vi "LSMcontroller_v62_updatedpointscan.vi"() -> ()   [LabVIEW 2015] (continued)
                            n96 = call "createdatafolder.vi"("timestamp in"=w2092) -> ("current data path"=w2093:path, "timestamp out"=w2091:timestamp)
                            n97 = local write "data dir"(w2093) -> ()
                          }
                        }
                        n98 = stacked-sequence {
                          tunnel: w2088 -> [_ w2100 _ _ _ _ _ _ _ _]
                          tunnel: [_ _ _ _ _ w2243 _ _ _ _] -> w2086
                          tunnel: [_ _ _ _ _ w2242 _ _ _ _] -> w2085
                          tunnel: [_ _ _ _ _ w2241 _ _ _ _] -> w2084
                          tunnel: [_ _ _ _ _ w2240 _ _ _ _] -> w2083
                          tunnel: [_ _ _ _ _ w2239 _ _ _ _] -> w2082
                          tunnel: [_ _ _ _ _ w2238 _ _ _ _] -> w2081
                          tunnel: [_ _ _ _ _ w2237 _ _ _ _] -> w2080
                          tunnel: [_ _ _ _ _ w2236 _ _ _ _] -> w2079
                          tunnel: [_ _ _ _ _ w2235 _ _ _ _] -> w2078
                          tunnel: [_ _ _ _ _ w2234 _ _ _ _] -> w2077
                          tunnel: [_ _ _ _ _ w2233 _ _ _ _] -> w2076
                          tunnel: [_ _ _ _ _ w2232 _ _ _ _] -> w2075
                          tunnel: [_ _ _ _ _ w2231 _ _ _ _] -> w2074
                          tunnel: [_ _ _ _ _ w2230 _ _ _ _] -> w2073
                          frame #0 {
                            n99 = local read "AI channels"() -> (w2099:i32[])
                            n100 = local read "CI channels"() -> (w2098:i32[])
                            n101 = call "2pparameters.vi"("command"="get") -> ("params out"=w2096:T10)  [unwired: 1 in]
                            n102 = Bundle By Name(cluster=w2096, "aAI"=w2099, "aCI"=w2098) -> (w2097:T10)
                            n103 = call "2pparameters.vi"("Params in"=w2097, "command"="set") -> ()  [unwired: 1 out]
                          }
                          frame #1 {
                            n104 = local read "Vy-min ref"() -> (w2104:dbl)
                            n105 = local read "Vy-max ref"() -> (w2105:dbl)
                            n106 = local read "Angle ref"() -> (w2103:dbl)
                            n107 = local read "Vx-min ref"() -> (w2106:dbl)
                            n108 = local write "counts"(0 ("counts")) -> ()
                            n109 = local write "graphtab"(T5."image" ("graphtab")) -> ()
                            n110 = local read "Vx-max ref"() -> (w2107:dbl)
                            n111 = property on="Stop" class="Bool (strict)"("Visible"=TRUE, "DisabledEnum"=T7."Enabled" ("Disabled")) -> ()  [unwired: 2 in, 2 out]
                            n112 = property on="Start" class="Bool (strict)"("Visible"=FALSE, "DisabledEnum"=T7."Disabled and Grayed Out" ("Disabled")) -> ()  [unwired: 2 in, 2 out]
                            n113 = script code="Xic=(ximax+ximin)./2;\nYic=(yimax+yimin)./2;\nximin=ximin-Xic;\nymin=ymin-Yic;\nxirmin=ximin.*cos(pi/180.*phi)+yimin.*sin(pi./180.*phi)+Xic;\nyirmin=-ximin.*sin(pi./180.*phi)+yimin.*cos(pi./180.*phi)+Yic;"("ximax"=w2107, "ximin"=w2106, "yimax"=w2105, "yimin"=w2104, "phi"=w2103) -> ("xirmin"=w2102:dbl, "yirmin"=w2101:dbl)  [unwired: 1 in, 1 out]
                            n114 = stacked-sequence {
                              tunnel: w2100 -> [_ w2132 _]
                              frame #0 {
                                n115 = local read "Measurement"() -> (w2114:T4)
                                n116 = case shown="\"X-Y-Z stack\"" w2114 {
                                frame "X-Y-t movie", Default {
                                n117 = call "2pparameters.vi"("command"="get") -> ("params out"=w2117:T10)  [unwired: 1 in]
                                n118 = Bundle By Name(cluster=w2117, "type"="X-Y-t movie") -> (w2115:T10)
                                n119 = call "2pparameters.vi"("Params in"=w2115, "command"="set") -> ()  [unwired: 1 out]
                                }
                                frame "X-Y-Z stack" {
                                n120 = call "2pparameters.vi"("command"="get") -> ("params out"=w2122:T10)  [unwired: 1 in]
                                n121 = Bundle By Name(cluster=w2122, "type"="X-Y-Z stack") -> (w2120:T10)
                                n122 = call "2pparameters.vi"("Params in"=w2120, "command"="set") -> ()  [unwired: 1 out]
                                }
                                frame "Lifetime (scan)" {
                                n123 = call "2pparameters.vi"("command"="get") -> ("params out"=w2127:T10)  [unwired: 1 in]
                                n124 = Bundle By Name(cluster=w2127, "type"="Lifetime (scan)") -> (w2125:T10)
                                n125 = call "2pparameters.vi"("Params in"=w2125, "command"="set") -> ()  [unwired: 1 out]
                                }
                                }
                              }
                              frame #1 {
                                n126 = Format Date/Time String(time format string (%c)="%Y%m%d", seconds (now)=w2132) -> (date/time string=w2131:string)  [unwired: 1 in]
                                n127 = Format Date/Time String(time format string (%c)="%H%M%S", seconds (now)=w2132) -> (date/time string=w2130:string)  [unwired: 1 in]
                                n128 = call "2pparameters.vi"("command"="get") -> ("params out"=w2136:T10)  [unwired: 1 in]
                                n129 = Bundle By Name(cluster=w2136, "date"=w2131, "time"=w2130) -> (w2135:T10)
                                n130 = call "2pparameters.vi"("Params in"=w2135, "command"="set") -> ()  [unwired: 1 out]
                              }
                              frame #2 {
                                n131 = call "configuration.vi"("command"="get") -> ("config out"=w2146:T11)  [unwired: 2 in, 1 out]
                                n132 = Unbundle By Name(w2146) -> ("CI names"=w2147:string[], "AI names"=w2148:string[])
                                n133 = call "2pparameters.vi"("command"="get") -> ("params out"=w2142:T10)  [unwired: 1 in]
                                n134 = Unbundle By Name(w2142) -> ("aCI"=w2143:i32[], "aAI"=w2144:i32[])
                                n135 = for {
                                tunnel: w2143 -> [w2158] mode=indexing
                                tunnel: w2147 -> [w2159]
                                tunnel: [w2157] -> w2149 mode=indexing
                                n136 = Index Array(array=w2159, index=w2158) -> (element=w2157:string)
                                }
                                n137 = for {
                                tunnel: w2144 -> [w2155] mode=indexing
                                tunnel: w2148 -> [w2156]
                                tunnel: [w2154] -> w2150 mode=indexing
                                n138 = Index Array(array=w2156, index=w2155) -> (element=w2154:string)
                                }
                                n139 = Build Array (concatenate)(w2149, w2150) -> (w2140:string[])
                                n140 = for {
                                tunnel: w2140 -> [w2152] mode=indexing
                                tunnel: [w2151] -> w2139 mode=indexing
                                i -> [w2153]
                                n141 = Bundle("String"=w2152, w2153) -> (w2151:cluster{"String":string, i32})  [unwired: 1 in]
                                }
                                n142 = property on="image1list" class="Ring (strict)"("StringsAndValues[]"=w2139) -> ()  [unwired: 2 in, 2 out]
                                n143 = property on="image2list" class="Ring (strict)"("StringsAndValues[]"=w2139) -> ()  [unwired: 2 in, 2 out]
                              }
                            }
                            n144 = call "setposition.vi"("Vy"=w2101, "Vx"=w2102) -> ()  [unwired: 1 in]
                          }
                          frame #2 {
                            n145 = call "X-array-databuffer.vi"("command"=enum16{"get", "set", "clear", "append"}."clear") -> ()  [unwired: 3 in, 2 out]
                            n146 = call "Y-array-databuffer.vi"("command"=enum16{"get", "set", "clear", "append"}."clear") -> ()  [unwired: 3 in, 2 out]
                            n147 = call "2pparameters.vi"("command"="get") -> ("params out"=w2162:T10)  [unwired: 1 in]
                            n148 = Unbundle By Name(w2162) -> ("autoshutter"=w2163:bool, "auto OD"=w2160:bool)
                            n149 = call "allAI-temp_img.vi"("command"=enum16{"get", "set", "clear", "append"}."clear") -> ()  [unwired: 3 in, 2 out]
                            n150 = case shown="True" w2160 {
                              frame False {
                              }
                              frame True {
                                n151 = call "configuration.vi"("command"="get") -> ("config out"=w2171:T11)  [unwired: 2 in, 1 out]
                                n152 = Unbundle By Name(w2171) -> ("image OD"=w2172:u16)
                                n153 = local read "ODfilt"() -> (w2169:u16)
                                n154 = call "filterwheelcontrol_nothorlabslib.vi"("Current OD filt"=w2169, "New ODfilt"=w2172) -> ()  [unwired: 1 in]
                              }
                            }
                            n155 = case shown="True" w2163 {
                              frame False {
                              }
                              frame True {
                                n156 = call "shuttercontrol.vi"("command"="close") -> ()  [unwired: 1 in, 1 out]
                              }
                            }
                            n157 = call "CH1-temp.vi"("command"=enum16{"get", "set", "clear", "add row"}."clear") -> ()  [unwired: 3 in, 2 out]
                            n158 = call "CH2-temp.vi"("command"=enum16{"get", "set", "clear", "add row"}."clear") -> ()  [unwired: 3 in, 2 out]
                          }
                          frame #3 {
                            n159 = local read "avpp"() -> (w2206:i32)
                            n160 = local read "Angle ref"() -> (w2205:dbl)
                            n161 = local read "ROI Type"() -> (w2204:u16)
                            n162 = local read "xpixels ref"() -> (w2201:i32)
                            n163 = local read "Vx-min ref"() -> (w2200:dbl)
                            n164 = local read "Vx-max ref"() -> (w2199:dbl)
                            n165 = local read "ypixels ref"() -> (w2197:i32)
                            n166 = local read "Vy-min ref"() -> (w2198:dbl)
                            n167 = local read "Vy-max ref"() -> (w2194:dbl)
                            n168 = local read "Sampling rate"() -> (w2188:dbl)
                            n169 = local read "finite samples"() -> (w2189:bool)
                            n170 = local read "continuous"() -> (w2192:bool)
                            n171 = local read "wavdet"() -> (w2193:bool)
                            n172 = local read "# of frames"() -> (w2191:i32)
                            n173 = local read "maxbufferAI"() -> (w2190:i32)
                            n174 = local read "Override AI buffer"() -> (w2174:bool)
                            n175 = call "2pparameters.vi"("command"="get") -> ("params out"=w2203:T10)  [unwired: 1 in]
                            n176 = Bundle By Name(cluster=w2203, "avpp"=w2206, "Angle Img"=w2205, "Xpixels Img"=w2201, "Vx-min Img"=w2200, "VX-max Img"=w2199, "Ypixels Img"=w2197, "Vy-min Img"=w2198, "Vy-max Img"=w2194, "srate"=w2188, "srate Img"=w2188, "finite"=w2189, "cont"=w2192, "wavdet"=w2193, "measpoints"=w2191, "maxbufferAI"=w2190, "Drawing Mode"=w2204, "Vz-reset"=0.0, "AIoverride"=w2174) -> (w2195:T10)
                            n177 = call "2pparameters.vi"("Params in"=w2195, "command"="set") -> ()  [unwired: 1 out]
                            n178 = local read "Vholding (mV)"() -> (w2177:sgl)
                            n179 = local read "Current Clamp"() -> (w2183:bool)
                            n180 = local read "Voltage Clamp"() -> (w2182:bool)
                            n181 = local read "OCgain"() -> (w2178:sgl)
                            n182 = local read "CC_ICgain"() -> (w2181:dbl)
                            n183 = local read "holdon"() -> (w2176:bool)
                            n184 = call "patchparameters.vi"("command"="get") -> ("Params out"=w2185:T13)  [unwired: 1 in]
                            n185 = Bundle By Name(cluster=w2185, "VC"=w2182, "CC"=w2183, "CC_icg (pA/mv)"=w2181, "VC_icg (mV/mV)"=sgl 10.0, "OCG (mV/pA)"=w2178, "OVG (mV/mV)"=0.1, "Vhold (mV)"=w2177, "holdon"=w2176) -> (w2184:T13)
                            n186 = call "patchparameters.vi"("Params in"=w2184, "command"="set") -> ()  [unwired: 1 out]
                          }
                          frame #4 {
                            # "Generate Waveforms for Scanning Mirrors"
                            n187 = call "2pparameters.vi"("command"="get") -> ("params out"=w2221:T10)  [unwired: 1 in]
                            n188 = Unbundle By Name(w2221) -> ("srate Img"=w2220:sgl, "Angle Img"=w2219:dbl, "VX-max Img"=w2218:dbl, "Vx-min Img"=w2217:dbl, "Xpixels Img"=w2216:i32, "Ypixels Img"=w2215:i32, "Vy-max Img"=w2214:dbl, "Vy-min Img"=w2213:dbl, "Drawing Mode"=w2212:u16)
                            n189 = call "ROI-databuffer.vi"("command"=enum16{"get", "set", "clear", "append"}."get") -> ("array out"=w2211:cluster{"x":sgl, "y":sgl}[])  [unwired: 4 in]
                            n190 = call "ScanningWaveform_v4.vi"("Vy-min"=w2213, "Vy-max"=w2214, "yPixels/tPixels"=w2215, "xPixels/rPixels"=w2216, "Vx-min"=w2217, "Vx-max"=w2218, "Drawing Mode"=w2212, "Angle"=w2219, "AOrate"=w2220, "Points"=w2211) -> ("numPixels"=w2207:dbl, "Y-WaveArray"=w2210:dbl[], "P"=w2208:dbl, "X-WaveArray"=w2209:dbl[])  [unwired: 6 in]
                            n191 = call "2pparameters.vi"("command"="get") -> ("params out"=w2229:T10)  [unwired: 1 in]
                            n192 = call "Y-array-databuffer.vi"("array in"=w2210, "command"=enum16{"get", "set", "clear", "append"}."set") -> ()  [unwired: 2 in, 2 out]
                            n193 = call "X-array-databuffer.vi"("array in"=w2209, "command"=enum16{"get", "set", "clear", "append"}."set") -> ()  [unwired: 2 in, 2 out]
                            n194 = Bundle By Name(cluster=w2229, "P"=w2208, "sAOxy"=w2207) -> (w2226:T10)
                            n195 = call "2pparameters.vi"("Params in"=w2226, "command"="set") -> ()  [unwired: 1 out]
                          }
                          frame #5 {
                            # "rem2Ps"
                            # "A2Ps"
                            # "Al"
                            # "Rl"
                            n196 = stacked-sequence {
                              seq-local: [w2248 _ _ _ _ _ _ _ _ _ _] -> [_ w2360 _ w2415 _ w2495 _ _ _ _ _]
                              seq-local: [w2249 _ _ _ _ _ _ _ _ _ _] -> [_ w2361 w2371 _ w2464 _ _ _ _ _ _]
                              seq-local: [_ _ w2370 _ _ _ _ _ _ _ _] -> [_ _ _ _ w2458 _ _ _ _ _ _]
                              seq-local: [_ _ _ w2414 _ _ _ _ _ _ _] -> [_ _ _ _ _ w2494 _ _ _ _ _]
                              seq-local: [w2245 _ _ _ _ _ _ _ _ _ _] -> [_ w2357 _ _ _ _ _ _ w2680 w2748 _]
                              seq-local: [w2244 _ _ _ _ _ _ _ _ _ _] -> [_ w2356 _ _ _ _ _ _ w2681 w2749 _]
                              seq-local: [w2251 _ _ _ _ _ _ _ _ _ _] -> [_ _ _ _ _ _ w2533 _ w2679 w2747 _]
                              seq-local: [w2247 _ _ _ _ _ _ _ _ _ _] -> [_ w2355 _ _ _ _ w2532 w2600 _ _ _]
                              seq-local: [w2246 _ _ _ _ _ _ _ _ _ _] -> [_ w2354 _ _ _ _ w2531 w2599 _ _ _]
                              seq-local: [w2250 _ _ _ _ _ _ _ _ _ _] -> [_ _ _ _ _ _ w2530 w2598 _ _ _]
                              tunnel: [_ _ w2369 _ _ _ _ _ _ _ _] -> w2242
                              tunnel: [_ _ w2368 _ _ _ _ _ _ _ _] -> w2241
                              tunnel: [w2249 _ _ _ _ _ _ _ _ _ _] -> w2243
                              tunnel: [w2248 _ _ _ _ _ _ _ _ _ _] -> w2240
                              tunnel: [_ _ _ w2413 _ _ _ _ _ _ _] -> w2239
                              tunnel: [_ _ _ w2412 _ _ _ _ _ _ _] -> w2238
                              tunnel: [w2247 _ _ _ _ _ _ _ _ _ _] -> w2237
                              tunnel: [w2246 _ _ _ _ _ _ _ _ _ _] -> w2236
                              tunnel: [_ _ _ _ _ _ w2529 _ _ _ _] -> w2235
                              tunnel: [_ _ _ _ _ _ _ w2597 _ _ _] -> w2234
                              tunnel: [w2245 _ _ _ _ _ _ _ _ _ _] -> w2233
                              tunnel: [w2244 _ _ _ _ _ _ _ _ _ _] -> w2232
                              tunnel: [_ _ _ _ _ _ _ _ w2678 _ _] -> w2231
                              tunnel: [_ _ _ _ _ _ _ _ _ w2746 _] -> w2230
                              frame #0 {
                                # "for a next version, give ome thought to\nthe possibilit of intermittently updating the\nwaveforms. it will have to be a calculation\nbased on speed of CPU and program on the one hand\nand length of measurement on the other. but then it should be possible, in principle, to \nupdate the waveform on the fly and that way cut up a longer measurement in smaller parts."
                                # "Y"
                                # "X"
                                n197 = stacked-sequence {
                                tunnel: [w2252 _ _ _] -> w2249
                                tunnel: [_ w2264 _ _] -> w2248
                                tunnel: [_ _ _ w2321] -> w2244
                                tunnel: [_ _ _ w2320] -> w2245
                                tunnel: [_ _ _ w2319] -> w2251
                                tunnel: [_ _ w2279 _] -> w2247
                                tunnel: [_ _ w2278 _] -> w2246
                                tunnel: [_ _ w2277 _] -> w2250
                                frame #0 {
                                n198 = call "configuration.vi"("command"="get") -> ("config out"=w2254:T11)  [unwired: 2 in, 1 out]
                                n199 = Unbundle By Name(w2254) -> ("Voltage to Xgalvo"=w2253:i32)
                                n200 = call "2pparameters.vi"("command"="get") -> ("params out"=w2258:T10)  [unwired: 1 in]
                                n201 = in-place {
                                in-place-border: w2253 -> [w2263]
                                in-place-border: [w2260] -> w2252
                                n202 = in-place-cluster #1(w2258) -> ("aAO"=w2262:u32[])
                                n203 = call "add channel to active arrayv2.vi"("line array in"=w2262, "line to add"=w2263) -> ("line array out"=w2261:u32[], "addition"=w2260:bool)  [unwired: 1 out]
                                n204 = in-place-cluster #1("aAO"=w2261) -> (w2256:T10)
                                }
                                n205 = call "2pparameters.vi"("Params in"=w2256, "command"="set") -> ()  [unwired: 1 out]
                                }
                                frame #1 {
                                n206 = call "configuration.vi"("command"="get") -> ("config out"=w2266:T11)  [unwired: 2 in, 1 out]
                                n207 = Unbundle By Name(w2266) -> ("Voltage to Ygalvo"=w2265:i32)
                                n208 = call "2pparameters.vi"("command"="get") -> ("params out"=w2270:T10)  [unwired: 1 in]
                                n209 = in-place {
                                in-place-border: w2265 -> [w2275]
                                in-place-border: [w2272] -> w2264
                                n210 = in-place-cluster #2(w2270) -> ("aAO"=w2274:u32[])
                                n211 = call "add channel to active arrayv2.vi"("line array in"=w2274, "line to add"=w2275) -> ("line array out"=w2273:u32[], "addition"=w2272:bool)  [unwired: 1 out]
                                n212 = in-place-cluster #2("aAO"=w2273) -> (w2268:T10)
                                }
                                n213 = call "2pparameters.vi"("Params in"=w2268, "command"="set") -> ()  [unwired: 1 out]
                                }
                                frame #2 {
                                n214 = call "2pparameters.vi"("command"="get") -> ("params out"=w2281:T10)  [unwired: 1 in]
                                n215 = Unbundle By Name(w2281) -> ("autoshutter"=w2280:bool, "wavdet"=w2276:bool)
                                n216 = case shown="True" w2280 {
                                tunnel: [w2286 w2306] -> w2279
                                tunnel: [w2285 FALSE ("removal")] -> w2278
                                tunnel: [w2284 w2304] -> w2277
                                tunnel: w2276 -> [w2283 _]
                                frame False {
                                n217 = case shown="False" w2283 {
                                tunnel: [FALSE ("addition") FALSE ("addition")] -> w2286
                                tunnel: [w2288 FALSE ("removal")] -> w2285
                                tunnel: [w2287 _] -> w2284
                                frame False {
                                n218 = call "configuration.vi"("command"="get") -> ("config out"=w2294:T11)  [unwired: 2 in, 1 out]
                                n219 = Unbundle By Name(w2294) -> ("2P shutter"=w2291:i32)
                                n220 = call "2pparameters.vi"("command"="get") -> ("params out"=w2292:T10)  [unwired: 1 in]
                                n221 = in-place {
                                in-place-border: w2291 -> [w2301]
                                in-place-border: [w2298] -> w2288
                                in-place-border: [w2297] -> w2287
                                n222 = in-place-cluster #3(w2292) -> ("aDO"=w2300:u32[])
                                n223 = call "remove channel from active arrayv2.vi"("line array in"=w2300, "line to remove"=w2301) -> ("line array out"=w2299:u32[], "removal"=w2298:bool, "index"=w2297:i32)
                                n224 = in-place-cluster #3("aDO"=w2299) -> (w2289:T10)
                                }
                                n225 = call "2pparameters.vi"("Params in"=w2289, "command"="set") -> ()  [unwired: 1 out]
                                }
                                frame True {
                                }
                                }
                                }
                                frame True {
                                n226 = call "configuration.vi"("command"="get") -> ("config out"=w2308:T11)  [unwired: 2 in, 1 out]
                                n227 = call "2pparameters.vi"("command"="get") -> ("params out"=w2312:T10)  [unwired: 1 in]
                                n228 = Unbundle By Name(w2308) -> ("2P shutter"=w2307:i32)
                                n229 = in-place {
                                in-place-border: w2307 -> [w2318]
                                in-place-border: [w2315] -> w2306
                                in-place-border: [w2314] -> w2304
                                n230 = in-place-cluster #4(w2312) -> ("aDO"=w2317:u32[])
                                n231 = call "add channel to active arrayv2.vi"("line array in"=w2317, "line to add"=w2318) -> ("line array out"=w2316:u32[], "addition"=w2315:bool, "index"=w2314:i32)
                                n232 = in-place-cluster #4("aDO"=w2316) -> (w2310:T10)
                                }
                                n233 = call "2pparameters.vi"("Params in"=w2310, "command"="set") -> ()  [unwired: 1 out]
                                }
                                }
                                }
                                frame #3 {
                                n234 = local read "Measurement"() -> (w2322:T4)
                                n235 = To Unsigned Long Integer(number=w2322) -> (unsigned 32bit integer=w2323:u32)
                                n236 = case shown="5..7" w2323 {
                                tunnel: [FALSE ("addition") w2341] -> w2321
                                tunnel: [w2326 FALSE ("removal")] -> w2320
                                tunnel: [w2324 w2339] -> w2319
                                frame 0..4, Default {
                                n237 = call "configuration.vi"("command"="get") -> ("config out"=w2332:T11)  [unwired: 2 in, 1 out]
                                n238 = Unbundle By Name(w2332) -> ("LT timestamp"=w2329:u32)
                                n239 = call "2pparameters.vi"("command"="get") -> ("params out"=w2330:T10)  [unwired: 1 in]
                                n240 = in-place {
                                in-place-border: w2329 -> [w2338]
                                in-place-border: [w2335] -> w2326
                                in-place-border: [w2334] -> w2324
                                n241 = in-place-cluster #5(w2330) -> ("aDO"=w2337:u32[])
                                n242 = call "remove channel from active arrayv2.vi"("line array in"=w2337, "line to remove"=w2338) -> ("line array out"=w2336:u32[], "removal"=w2335:bool, "index"=w2334:i32)
                                n243 = in-place-cluster #5("aDO"=w2336) -> (w2327:T10)
                                }
                                n244 = call "2pparameters.vi"("Params in"=w2327, "command"="set") -> ()  [unwired: 1 out]
                                }
                                frame 5..7 {
                                n245 = call "configuration.vi"("command"="get") -> ("config out"=w2347:T11)  [unwired: 2 in, 1 out]
                                n246 = Unbundle By Name(w2347) -> ("LT timestamp"=w2344:u32)
                                n247 = call "2pparameters.vi"("command"="get") -> ("params out"=w2345:T10)  [unwired: 1 in]
                                n248 = in-place {
                                in-place-border: w2344 -> [w2353]
                                in-place-border: [w2350] -> w2341
                                in-place-border: [w2349] -> w2339
                                n249 = in-place-cluster #6(w2345) -> ("aDO"=w2352:u32[])
                                n250 = call "add channel to active arrayv2.vi"("line array in"=w2352, "line to add"=w2353) -> ("line array out"=w2351:u32[], "addition"=w2350:bool, "index"=w2349:i32)
                                n251 = in-place-cluster #6("aDO"=w2351) -> (w2342:T10)
                                }
                                n252 = call "2pparameters.vi"("Params in"=w2342, "command"="set") -> ()  [unwired: 1 out]
                                }
                                }
                                }
                                }
                              }
                              frame #1 {
                                n253 = Or(x=w2360, y=w2361) -> (x .or. y?=w2359:bool)
                                n254 = case shown="True" w2359 {
                                frame False {
                                }
                                frame True {
                                # "update GUI"
                                n255 = call "Used AO lines.vi"() -> ("used AO names"=w2365:string[], "used AO lines"=w2367:tag[])  [unwired: 2 in]
                                n256 = control-ref of="Analog Lines Plot"() -> (w2366:refnum<vi>)
                                n257 = local write "Analog Used Lines"(w2367) -> ()
                                n258 = local write "Analog Used Names"(w2365) -> ()
                                n259 = call "prepAOWaveplot.vi"("WaveformGraph in"=w2366, "Analog Used Names"=w2365) -> ()  [unwired: 1 in]
                                }
                                }
                                n260 = Compound Arithmetic op=OR(w2357, w2356, w2355, w2354) -> (w2358:bool)
                                n261 = case shown="True" w2358 {
                                frame False {
                                }
                                frame True {
                                n262 = control-ref of="Digital Lines Plot"() -> (w2362:refnum<vi>)
                                n263 = call "Used DO lines.vi"() -> ("used DO names"=w2363:string[], "used DO lines"=w2364:tag[])  [unwired: 2 in]
                                n264 = local write "Digital Used Lines"(w2364) -> ()
                                n265 = local write "Digital Used Names"(w2363) -> ()
                                n266 = call "prepDOWaveplot.vi"("DigitalGraph in"=w2362, "used DO names"=w2363) -> ()  [unwired: 1 in]
                                }
                                }
                              }
                              frame #2 {
                                n267 = case shown="False" w2371 {
                                tunnel: [w2374 w2395] -> w2370
                                tunnel: [w2373 w2393] -> w2369
                                tunnel: [w2372 _] -> w2368
                                frame False {
                                n268 = stacked-sequence {
                                seq-local: [w2376 _] -> [_ w2389]
                                tunnel: [w2376 _] -> w2374
                                tunnel: [w2379 _] -> w2373
                                tunnel: [w2375 _] -> w2372
                                frame #0 {
                                n269 = call "configuration.vi"("command"="get") -> ("config out"=w2387:T11)  [unwired: 2 in, 1 out]
                                n270 = call "waveformparamsv2.vi"("command"="get") -> ("Params out"=w2381:T14)  [unwired: 4 in, 2 out]
                                n271 = Unbundle By Name(w2387) -> ("Voltage to Xgalvo"=w2388:i32)
                                n272 = call "2pparameters.vi"("command"="get") -> ("params out"=w2384:T10)  [unwired: 1 in]
                                n273 = Unbundle By Name(w2381) -> ("AO parameters"=w2380:T15)
                                n274 = Unbundle By Name(w2384) -> ("aAO"=w2385:u32[])
                                n275 = call "waveformsAObuffer.vi"("command"="get") -> ("AO wf out"=w2377:waveform(dbl)[])  [unwired: 1 in]
                                n276 = Search 1D Array(1D array=w2385, element=w2388) -> (index of element=w2376:i32)  [unwired: 1 in]
                                n277 = Index Array(array=w2377, index=w2376) -> (element=w2375:waveform(dbl))
                                n278 = Index Array(array=w2380, index=w2376) -> (element=w2379:T16)
                                }
                                frame #1 {
                                w2390 = 0.0 ("Step size (V)")
                                n279 = local read "Sampling rate"() -> (w2391:dbl)
                                n280 = call "replace AO XYwfparam.vi"("Baseline (V)"=w2390, "Start amplitude (V)"=w2390, "Cycles"=w2390, "Repeats"=w2390, "index of AO wave"=w2389, "Step size (V)"=w2390, "DC (%)"=w2390, "Sampling frequency (Hz)"=w2391, "Period (ms)"=w2390, "Cycle length (s)"=w2390, "Pulses"=w2390, "padding value"=w2390, "Matlab wave name"=path "xwave") -> ()  [unwired: 3 in]
                                }
                                }
                                }
                                frame True {
                                w2394 = 0.0 ("Repeats")
                                n281 = local read "Sampling rate"() -> (w2403:dbl)
                                n282 = call "2pparameters.vi"("command"="get") -> ("params out"=w2397:T10)  [unwired: 1 in]
                                n283 = call "configuration.vi"("command"="get") -> ("config out"=w2400:T11)  [unwired: 2 in, 1 out]
                                n284 = call "waveformparamsv2.vi"("command"="get") -> ("Params out"=w2409:T14)  [unwired: 4 in, 2 out]
                                n285 = Unbundle By Name(w2400) -> ("Voltage to Xgalvo"=w2401:i32)
                                n286 = Unbundle By Name(w2409) -> ("AO parameters"=w2406:T15)
                                n287 = Unbundle By Name(w2397) -> ("aAO"=w2398:u32[])
                                n288 = Search 1D Array(1D array=w2398, element=w2401) -> (index of element=w2395:i32)  [unwired: 1 in]
                                n289 = Index Array(array=w2406, index=0) -> (element=w2407:T16)
                                n290 = Bundle By Name(cluster=w2407, "AOtab"=-1.0 ("Repeats"), "Repeats"=w2394, "Cycles"=w2394, "Start amplitude (V)"=w2394, "Baseline (V)"=w2394, "Step size (V)"=w2394, "DC (%)"=w2394, "Sampling frequency (Hz)"=w2403, "Period (ms)"=w2394, "Offset (V)"=w2394, "Amplitude (V)"=w2394, "Frequency"=w2394, "Tri Repeats"=w2394, "phase shift (ms)"=w2394, "Pulses"=w2394, "Matlab wave file"=path "xwave", "padding value"=w2394) -> (w2393:T16)
                                n291 = Build Array(w2393) -> (w2404:T15)
                                n292 = call "waveformparamsv2.vi"("command"="add AO", "add AO"=w2404) -> ()  [unwired: 3 in, 3 out]
                                }
                                }
                              }
                              frame #3 {
                                n293 = case shown="False" w2415 {
                                tunnel: [w2418 w2439] -> w2414
                                tunnel: [w2417 w2437] -> w2413
                                tunnel: [w2416 _] -> w2412
                                frame False {
                                n294 = stacked-sequence {
                                seq-local: [w2420 _] -> [_ w2433]
                                tunnel: [w2420 _] -> w2418
                                tunnel: [w2423 _] -> w2417
                                tunnel: [w2419 _] -> w2416
                                frame #0 {
                                n295 = call "configuration.vi"("command"="get") -> ("config out"=w2431:T11)  [unwired: 2 in, 1 out]
                                n296 = call "waveformparamsv2.vi"("command"="get") -> ("Params out"=w2425:T14)  [unwired: 4 in, 2 out]
                                n297 = Unbundle By Name(w2431) -> ("Voltage to Ygalvo"=w2432:i32)
                                n298 = call "2pparameters.vi"("command"="get") -> ("params out"=w2428:T10)  [unwired: 1 in]
                                n299 = Unbundle By Name(w2425) -> ("AO parameters"=w2424:T15)
                                n300 = Unbundle By Name(w2428) -> ("aAO"=w2429:u32[])
                                n301 = call "waveformsAObuffer.vi"("command"="get") -> ("AO wf out"=w2421:waveform(dbl)[])  [unwired: 1 in]
                                n302 = Search 1D Array(1D array=w2429, element=w2432) -> (index of element=w2420:i32)  [unwired: 1 in]
                                n303 = Index Array(array=w2421, index=w2420) -> (element=w2419:waveform(dbl))
                                n304 = Index Array(array=w2424, index=w2420) -> (element=w2423:T16)
                                }
                                frame #1 {
                                w2434 = 0.0 ("Step size (V)")
                                n305 = local read "Sampling rate"() -> (w2435:dbl)
                                n306 = call "replace AO XYwfparam.vi"("Baseline (V)"=w2434, "Start amplitude (V)"=w2434, "Cycles"=w2434, "Repeats"=w2434, "index of AO wave"=w2433, "Step size (V)"=w2434, "DC (%)"=w2434, "Sampling frequency (Hz)"=w2435, "Period (ms)"=w2434, "Cycle length (s)"=w2434, "Pulses"=w2434, "padding value"=w2434, "Matlab wave name"=path "ywave") -> ()  [unwired: 3 in]
                                }
                                }
                                }
                                frame True {
                                w2438 = 0.0 ("Repeats")
                                n307 = local read "Sampling rate"() -> (w2448:dbl)
                                n308 = call "2pparameters.vi"("command"="get") -> ("params out"=w2441:T10)  [unwired: 1 in]
                                n309 = call "configuration.vi"("command"="get") -> ("config out"=w2444:T11)  [unwired: 2 in, 1 out]
                                n310 = call "waveformparamsv2.vi"("command"="get") -> ("Params out"=w2454:T14)  [unwired: 4 in, 2 out]
                                n311 = Unbundle By Name(w2444) -> ("Voltage to Ygalvo"=w2445:i32)
                                n312 = Unbundle By Name(w2454) -> ("AO parameters"=w2451:T15)
                                n313 = Unbundle By Name(w2441) -> ("aAO"=w2442:u32[])
                                n314 = Search 1D Array(1D array=w2442, element=w2445) -> (index of element=w2439:i32)  [unwired: 1 in]
                                n315 = Index Array(array=w2451, index=0) -> (element=w2452:T16)
                                n316 = Bundle By Name(cluster=w2452, "AOtab"=-1.0 ("Repeats"), "Repeats"=w2438, "Cycles"=w2438, "Start amplitude (V)"=w2438, "Baseline (V)"=w2438, "Step size (V)"=w2438, "DC (%)"=w2438, "Sampling frequency (Hz)"=w2448, "Period (ms)"=w2438, "Offset (V)"=w2438, "Amplitude (V)"=w2438, "Frequency"=w2438, "Tri Repeats"=w2438, "phase shift (ms)"=w2438, "Pulses"=w2438, "Matlab wave file"=path "ywave", "padding value"=w2438) -> (w2437:T16)
                                n317 = Build Array(w2437) -> (w2449:T15)
                                n318 = call "waveformparamsv2.vi"("command"="add AO", "add AO"=w2449) -> ()  [unwired: 3 in, 3 out]
                                }
                                }
                              }
                              frame #4 {
                                n319 = call "2pparameters.vi"("command"="get") -> ("params out"=w2461:T10)  [unwired: 1 in]
                                n320 = Unbundle By Name(w2461) -> ("wavdet"=w2460:bool, "sAOxy"=w2457:i32, "refwfsize"=w2456:dbl, "srate Img"=w2459:sgl)
                                n321 = case shown="False" w2460 {
                                tunnel: [w2465 w2475] -> w2463
                                tunnel: w2459 -> [w2466 w2477]
                                tunnel: w2457 -> [_ w2473]
                                tunnel: w2456 -> [_ w2472]
                                frame False {
                                n322 = call "X-array-databuffer.vi"("command"=enum16{"get", "set", "clear", "append"}."get") -> ("array out"=w2469:dbl[])  [unwired: 3 in, 1 out]
                                n323 = Reciprocal(x=w2466) -> (1/x=w2467:sgl)
                                n324 = Bundle By Name("Y"=w2469, "dt"=w2467) -> (w2465:waveform(dbl))  [unwired: 1 in]
                                }
                                frame True {
                                n325 = To Double Precision Float(number=w2473) -> (double precision float=w2474:dbl)
                                n326 = Divide(x=w2472, y=w2474) -> (x/y=w2470:dbl)
                                n327 = Round Toward +Infinity(x=w2470) -> (ceil(x): smallest int >= x=w2471:dbl)
                                n328 = call "X-array-databuffer.vi"("command"=enum16{"get", "set", "clear", "append"}."get") -> ("array out"=w2479:dbl[])  [unwired: 3 in, 1 out]
                                n329 = Reciprocal(x=w2477) -> (1/x=w2478:sgl)
                                n330 = for {
                                N: w2471 -> [_]
                                tunnel: w2479 -> [w2481]
                                tunnel: [w2481] -> w2476 mode=concatenating
                                }
                                n331 = Bundle By Name("Y"=w2476, "dt"=w2478) -> (w2475:waveform(dbl))  [unwired: 1 in]
                                }
                                }
                                n332 = case shown="False" w2464 {
                                tunnel: w2463 -> [w2483 w2489]
                                tunnel: w2458 -> [w2484 _]
                                frame False {
                                n333 = call "waveformsAObuffer.vi"("command"="get") -> ("AO wf out"=w2487:waveform(dbl)[])  [unwired: 1 in]
                                n334 = Replace Array Subset(array=w2487, new element=w2483, index=w2484) -> (w2482:waveform(dbl)[])
                                n335 = call "waveformsAObuffer.vi"("AO wf in"=w2482, "command"="set") -> ()  [unwired: 1 out]
                                }
                                frame True {
                                n336 = call "waveformsAObuffer.vi"("command"="get") -> ("AO wf out"=w2491:waveform(dbl)[])  [unwired: 1 in]
                                n337 = Build Array (concatenate)(w2491, w2489) -> (w2488:waveform(dbl)[])
                                n338 = call "waveformsAObuffer.vi"("AO wf in"=w2488, "command"="set") -> ()  [unwired: 1 out]
                                }
                                }
                              }
                              frame #5 {
                                n339 = call "2pparameters.vi"("command"="get") -> ("params out"=w2503:T10)  [unwired: 1 in]
                                n340 = Unbundle By Name(w2503) -> ("wavdet"=w2502:bool, "sAOxy"=w2500:i32, "refwfsize"=w2501:dbl, "srate Img"=w2496:sgl)
                                n341 = To Double Precision Float(number=w2500) -> (double precision float=w2499:dbl)
                                n342 = Divide(x=w2501, y=w2499) -> (x/y=w2498:dbl)
                                n343 = Round Toward +Infinity(x=w2498) -> (ceil(x): smallest int >= x=w2497:dbl)
                                n344 = case shown="True" w2502 {
                                tunnel: [w2507 w2512] -> w2493
                                tunnel: w2497 -> [_ w2516]
                                tunnel: w2496 -> [w2508 w2514]
                                frame False {
                                n345 = call "Y-array-databuffer.vi"("command"=enum16{"get", "set", "clear", "append"}."get") -> ("array out"=w2505:dbl[])  [unwired: 3 in, 1 out]
                                n346 = Reciprocal(x=w2508) -> (1/x=w2509:sgl)
                                n347 = Bundle By Name("Y"=w2505, "dt"=w2509) -> (w2507:waveform(dbl))  [unwired: 1 in]
                                }
                                frame True {
                                n348 = call "Y-array-databuffer.vi"("command"=enum16{"get", "set", "clear", "append"}."get") -> ("array out"=w2510:dbl[])  [unwired: 3 in, 1 out]
                                n349 = Reciprocal(x=w2514) -> (1/x=w2515:sgl)
                                n350 = for {
                                N: w2516 -> [_]
                                tunnel: w2510 -> [w2517]
                                tunnel: [w2517] -> w2513 mode=concatenating
                                }
                                n351 = Bundle By Name("Y"=w2513, "dt"=w2515) -> (w2512:waveform(dbl))  [unwired: 1 in]
                                }
                                }
                                n352 = case shown="False" w2495 {
                                tunnel: w2493 -> [w2520 w2525]
                                tunnel: w2494 -> [w2521 _]
                                frame False {
                                n353 = call "waveformsAObuffer.vi"("command"="get") -> ("AO wf out"=w2523:waveform(dbl)[])  [unwired: 1 in]
                                n354 = Replace Array Subset(array=w2523, new element=w2520, index=w2521) -> (w2518:waveform(dbl)[])
                                n355 = call "waveformsAObuffer.vi"("AO wf in"=w2518, "command"="set") -> ()  [unwired: 1 out]
                                }
                                frame True {
                                n356 = call "waveformsAObuffer.vi"("command"="get") -> ("AO wf out"=w2527:waveform(dbl)[])  [unwired: 1 in]
                                n357 = Build Array (concatenate)(w2527, w2525) -> (w2524:waveform(dbl)[])
                                n358 = call "waveformsAObuffer.vi"("AO wf in"=w2524, "command"="set") -> ()  [unwired: 1 out]
                                }
                                }
                              }
                              frame #6 {
                                n359 = Build Array(w2532, w2531) -> (w2535:bool[])
                                n360 = Boolean Array To Number(Boolean array=w2535) -> (number=w2534:u32)
                                n361 = case shown="0" w2534 {
                                tunnel: w2533 -> [_ _ _ _]
                                tunnel: w2530 -> [_ w2558 _ w2571]
                                tunnel: [_ w2557 _ w2568] -> w2529
                                frame 1 {
                                w2545 = 0.0 ("DOtab")
                                n362 = call "2pparameters.vi"("command"="get") -> ("params out"=w2542:T10)  [unwired: 1 in]
                                n363 = call "waveformparamsv2.vi"("command"="get") -> ("Params out"=w2553:T14)  [unwired: 4 in, 2 out]
                                n364 = Unbundle By Name(w2553) -> ("DO parameters"=w2551:T17)
                                n365 = Unbundle By Name(w2542) -> ("srate"=w2538:sgl, "sAOxy"=w2541:i32)
                                n366 = To Double Precision Float(number=w2538) -> (double precision float=w2536:dbl)
                                n367 = To Double Precision Float(number=w2538) -> (double precision float=w2537:dbl)
                                n368 = To Double Precision Float(number=w2541) -> (double precision float=w2540:dbl)
                                n369 = Divide(x=w2537, y=w2540) -> (x/y=w2539:dbl)
                                n370 = Index Array(array=w2551, index=0) -> (element=w2550:T18)
                                n371 = Bundle By Name(cluster=w2550, "Digital DC (%)"=100.0, "Digital phase"=w2545, "Digital Freq (Hz)"=w2539, "Sampling frequency (Hz)"=w2536, "Digital time offset (s)"=w2545, "padding value"=0.0, "matlab wave file"=path "2Pshutter", "DOtab"=0.0) -> (w2548:T18)
                                n372 = Build Array(w2548) -> (w2547:T17)
                                n373 = call "waveformparamsv2.vi"("command"="add DO", "add DO"=w2547) -> ()  [unwired: 3 in, 3 out]
                                }
                                frame 2 {
                                n374 = call "waveformparamsv2.vi"("command"="get") -> ("Params out"=w2560:T14)  [unwired: 4 in, 2 out]
                                n375 = in-place {
                                in-place-border: w2558 -> [w2564]
                                in-place-border: [w2563] -> w2557
                                n376 = in-place-cluster #7(w2560) -> ("DO parameters"=w2566:T17)
                                n377 = Delete From Array(array=w2566, length=1, index=w2564) -> (deleted portion=w2563:T17, array with subset deleted=w2565:T17)
                                n378 = in-place-cluster #7("DO parameters"=w2565) -> (w2559:T14)
                                }
                                n379 = call "waveformparamsv2.vi"("command"="set", "Params in"=w2559) -> ()  [unwired: 3 in, 3 out]
                                }
                                frame 3, Default {
                                }
                                frame 0 {
                                n380 = call "2pparameters.vi"("command"="get") -> ("params out"=w2573:T10)  [unwired: 1 in]
                                n381 = Unbundle By Name(w2573) -> ("wavdet"=w2570:bool, "autoshutter"=w2572:bool)
                                n382 = case shown="True" w2572 {
                                tunnel: w2571 -> [_ w2577]
                                tunnel: w2570 -> [_ w2576]
                                tunnel: [_ w2575] -> w2569
                                frame False {
                                }
                                frame True {
                                n383 = case shown="False" w2576 {
                                tunnel: w2577 -> [w2579 _]
                                tunnel: [w2578 _] -> w2575
                                frame False {
                                n384 = stacked-sequence {
                                tunnel: w2579 -> [w2581 w2595]
                                tunnel: [w2580 _] -> w2578
                                frame #0 {
                                n385 = call "waveformparamsv2.vi"("command"="get") -> ("Params out"=w2583:T14)  [unwired: 4 in, 2 out]
                                n386 = Unbundle By Name(w2583) -> ("DO parameters"=w2582:T17)
                                n387 = Index Array(array=w2582, index=w2581) -> (element=w2580:T18)
                                }
                                frame #1 {
                                w2594 = 0.0 ("padding value")
                                n388 = call "2pparameters.vi"("command"="get") -> ("params out"=w2592:T10)  [unwired: 1 in]
                                n389 = Unbundle By Name(w2592) -> ("srate"=w2589:sgl, "sAOxy"=w2591:i32)
                                n390 = To Double Precision Float(number=w2589) -> (double precision float=w2587:dbl)
                                n391 = To Double Precision Float(number=w2589) -> (double precision float=w2588:dbl)
                                n392 = To Double Precision Float(number=w2591) -> (double precision float=w2590:dbl)
                                n393 = Divide(x=w2588, y=w2590) -> (x/y=w2586:dbl)
                                n394 = call "replace DO wf param.vi"("Digital Freq (Hz)"=w2586, "Digital DC (%)"=100.0, "Digital phase"=w2594, "Sampling frequency (Hz)"=w2587, "Digital time offset (s)"=w2594, "index of DO wave"=w2595, "padding value"=w2594, "matlab wave file"=path "2Pshutter" ("matlab wave number")) -> ()  [unwired: 3 in]
                                }
                                }
                                }
                                frame True {
                                }
                                }
                                }
                                }
                                n395 = Build Array(w2569) -> (w2568:T17)
                                }
                                }
                              }
                              frame #7 {
                                n396 = Build Array(w2600, w2599) -> (w2602:bool[])
                                n397 = Boolean Array To Number(Boolean array=w2602) -> (number=w2601:u32)
                                n398 = case shown="2" w2601 {
                                tunnel: w2598 -> [_ w2644 _ w2651]
                                tunnel: [_ w2643 _ w2649] -> w2597
                                frame 1 {
                                n399 = call "2pparameters.vi"("command"="get") -> ("params out"=w2609:T10)  [unwired: 1 in]
                                n400 = Unbundle By Name(w2609) -> ("wavdet"=w2610:bool, "sAOxy"=w2612:i32, "refwfsize"=w2613:dbl, "srate Img"=w2611:sgl)
                                n401 = call "waveformsDObuffer.vi"("command"="get") -> ("DO wf out"=w2605:digitalwaveform[])  [unwired: 1 in]
                                n402 = case shown="False" w2610 {
                                tunnel: [w2618 w2628] -> w2607
                                tunnel: w2611 -> [w2623 w2639]
                                tunnel: w2612 -> [w2617 w2632]
                                tunnel: w2613 -> [_ w2636]
                                frame False {
                                w2621 = u16 0 items=["unsigned binary", "offset binary", "2's complement"] ("data format (offset binary)")
                                n403 = Initialize Array(sgl 1.0, w2617) -> (w2614:sgl[])
                                n404 = Reciprocal(x=w2623) -> (1/x=w2624:sgl)
                                n405 = Bundle By Name("Y"=w2614, "dt"=w2624) -> (w2619:waveform(sgl))  [unwired: 1 in]
                                n406 = call-poly <vilib>:"Analog to Digital.vi"("data format (offset binary)"=w2621, "compress digital (T)"=TRUE, "full-scale range (pk-pk)"=1.0, "resolution (16 bit)"=1, "analog waveform"=w2619) -> ("digital waveform"=w2618:digitalwaveform)  [unwired: 3 in, 3 out]
                                }
                                frame True {
                                w2631 = u16 0 items=["unsigned binary", "offset binary", "2's complement"] ("data format (offset binary)")
                                n407 = To Double Precision Float(number=w2632) -> (double precision float=w2637:dbl)
                                n408 = Initialize Array(sgl 1.0, w2632) -> (w2625:sgl[])
                                n409 = Divide(x=w2636, y=w2637) -> (x/y=w2634:dbl)
                                n410 = Round Toward +Infinity(x=w2634) -> (ceil(x): smallest int >= x=w2635:dbl)
                                n411 = for {
                                N: w2635 -> [_]
                                tunnel: w2625 -> [w2641]
                                tunnel: [w2641] -> w2638 mode=concatenating
                                }
                                n412 = Reciprocal(x=w2639) -> (1/x=w2640:sgl)
                                n413 = Bundle By Name("Y"=w2638, "dt"=w2640) -> (w2629:waveform(sgl))  [unwired: 1 in]
                                n414 = call-poly <vilib>:"Analog to Digital.vi"("data format (offset binary)"=w2631, "compress digital (T)"=TRUE, "full-scale range (pk-pk)"=1.0, "resolution (16 bit)"=1, "analog waveform"=w2629) -> ("digital waveform"=w2628:digitalwaveform)  [unwired: 3 in, 3 out]
                                }
                                }
                                n415 = Build Array (concatenate)(w2605, w2607) -> (w2603:digitalwaveform[])
                                n416 = call "waveformsDObuffer.vi"("DO wf in"=w2603, "command"="set") -> ()  [unwired: 1 out]
                                }
                                frame 2 {
                                n417 = call "waveformsDObuffer.vi"("command"="get") -> ("DO wf out"=w2646:digitalwaveform[])  [unwired: 1 in]
                                n418 = Delete From Array(array=w2646, length=1, index=w2644) -> (deleted portion=w2643:digitalwaveform[], array with subset deleted=w2642:digitalwaveform[])
                                n419 = call "waveformsDObuffer.vi"("DO wf in"=w2642, "command"="set") -> ()  [unwired: 1 out]
                                }
                                frame 3, Default {
                                }
                                frame 0 {
                                n420 = call "2pparameters.vi"("command"="get") -> ("params out"=w2653:T10)  [unwired: 1 in]
                                n421 = Unbundle By Name(w2653) -> ("autoshutter"=w2652:bool, "wavdet"=w2650:bool)
                                n422 = case shown="True" w2652 {
                                tunnel: w2651 -> [_ w2657]
                                tunnel: w2650 -> [_ w2656]
                                tunnel: [_ w2655] -> w2649
                                frame False {
                                }
                                frame True {
                                n423 = case shown="False" w2656 {
                                tunnel: w2657 -> [w2661 _]
                                tunnel: [w2659 _] -> w2655
                                frame False {
                                w2668 = u16 0 items=["unsigned binary", "offset binary", "2's complement"] ("data format (offset binary)")
                                n424 = call "2pparameters.vi"("command"="get") -> ("params out"=w2675:T10)  [unwired: 1 in]
                                n425 = Unbundle By Name(w2675) -> ("sAOxy"=w2677:i32, "srate Img"=w2676:sgl)
                                n426 = call "waveformsDObuffer.vi"("command"="get") -> ("DO wf out"=w2662:digitalwaveform[])  [unwired: 1 in]
                                n427 = Index Array(array=w2662, index=w2661) -> (element=w2660:digitalwaveform)
                                n428 = Build Array(w2660) -> (w2659:digitalwaveform[])
                                n429 = Initialize Array(sgl 1.0, w2677) -> (w2663:sgl[])
                                n430 = Reciprocal(x=w2676) -> (1/x=w2670:sgl)
                                n431 = Bundle By Name("Y"=w2663, "dt"=w2670) -> (w2666:waveform(sgl))  [unwired: 1 in]
                                n432 = call-poly <vilib>:"Analog to Digital.vi"("data format (offset binary)"=w2668, "compress digital (T)"=TRUE, "full-scale range (pk-pk)"=1.0, "resolution (16 bit)"=1, "analog waveform"=w2666) -> ("digital waveform"=w2673:digitalwaveform)  [unwired: 3 in, 3 out]
                                n433 = Replace Array Subset(array=w2662, new element=w2673, index=w2661) -> (w2658:digitalwaveform[])
                                n434 = call "waveformsDObuffer.vi"("DO wf in"=w2658, "command"="set") -> ()  [unwired: 1 out]
                                }
                                frame True {
                                }
                                }
                                }
                                }
                                }
                                }
                              }
                              frame #8 {
                                n435 = Build Array(w2681, w2680) -> (w2683:bool[])
                                n436 = Boolean Array To Number(Boolean array=w2683) -> (number=w2682:u32)
                                n437 = case shown="0" w2682 {
                                tunnel: w2679 -> [_ w2709 _ w2721]
                                tunnel: [_ w2708 _ w2719] -> w2678
                                frame 1 {
                                w2696 = 0.0 ("DOtab")
                                n438 = call "2pparameters.vi"("command"="get") -> ("params out"=w2694:T10)  [unwired: 1 in]
                                n439 = call "waveformparamsv2.vi"("command"="get") -> ("Params out"=w2704:T14)  [unwired: 4 in, 2 out]
                                n440 = Unbundle By Name(w2704) -> ("DO parameters"=w2702:T17)
                                n441 = Unbundle By Name(w2694) -> ("srate"=w2691:sgl, "sAOxy"=w2693:i32)
                                n442 = To Double Precision Float(number=w2691) -> (double precision float=w2689:dbl)
                                n443 = To Double Precision Float(number=w2691) -> (double precision float=w2690:dbl)
                                n444 = To Double Precision Float(number=w2693) -> (double precision float=w2685:dbl)
                                n445 = Divide(x=w2690, y=w2685) -> (x/y=w2692:dbl)
                                n446 = Index Array(array=w2702, index=0) -> (element=w2701:T18)
                                n447 = Divide(x=1.0 ("Digital DC (%)"), y=w2685) -> (x/y=w2687:dbl)
                                n448 = Multiply(x=100.0, y=w2687) -> (x*y=w2684:dbl)
                                n449 = Bundle By Name(cluster=w2701, "Digital DC (%)"=w2684, "Digital phase"=w2696, "Digital Freq (Hz)"=w2692, "Sampling frequency (Hz)"=w2689, "Digital time offset (s)"=w2696, "padding value"=0.0, "matlab wave file"=path "LT", "DOtab"=0.0) -> (w2699:T18)
                                n450 = Build Array(w2699) -> (w2698:T17)
                                n451 = call "waveformparamsv2.vi"("command"="add DO", "add DO"=w2698) -> ()  [unwired: 3 in, 3 out]
                                }
                                frame 2 {
                                n452 = call "waveformparamsv2.vi"("command"="get") -> ("Params out"=w2711:T14)  [unwired: 4 in, 2 out]
                                n453 = in-place {
                                in-place-border: w2709 -> [w2715]
                                in-place-border: [w2714] -> w2708
                                n454 = in-place-cluster #8(w2711) -> ("DO parameters"=w2717:T17)
                                n455 = Delete From Array(array=w2717, length=1, index=w2715) -> (deleted portion=w2714:T17, array with subset deleted=w2716:T17)
                                n456 = in-place-cluster #8("DO parameters"=w2716) -> (w2710:T14)
                                }
                                n457 = call "waveformparamsv2.vi"("command"="set", "Params in"=w2710) -> ()  [unwired: 3 in, 3 out]
                                }
                                frame 3, Default {
                                }
                                frame 0 {
                                n458 = local read "Measurement"() -> (w2723:T4)
                                n459 = To Unsigned Long Integer(number=w2723) -> (unsigned 32bit integer=w2722:u32)
                                n460 = case shown="5..7" w2722 {
                                tunnel: w2721 -> [_ w2725]
                                tunnel: [_ w2724] -> w2720
                                frame 0..4, Default {
                                }
                                frame 5..7 {
                                n461 = stacked-sequence {
                                tunnel: w2725 -> [w2727 w2736]
                                tunnel: [w2726 _] -> w2724
                                frame #0 {
                                n462 = call "waveformparamsv2.vi"("command"="get") -> ("Params out"=w2729:T14)  [unwired: 4 in, 2 out]
                                n463 = Unbundle By Name(w2729) -> ("DO parameters"=w2730:T17)
                                n464 = Index Array(array=w2730, index=w2727) -> (element=w2726:T18)
                                }
                                frame #1 {
                                w2744 = 0.0 ("padding value")
                                n465 = call "2pparameters.vi"("command"="get") -> ("params out"=w2742:T10)  [unwired: 1 in]
                                n466 = Unbundle By Name(w2742) -> ("srate"=w2740:sgl, "sAOxy"=w2741:i32)
                                n467 = To Double Precision Float(number=w2740) -> (double precision float=w2738:dbl)
                                n468 = To Double Precision Float(number=w2740) -> (double precision float=w2739:dbl)
                                n469 = To Double Precision Float(number=w2741) -> (double precision float=w2734:dbl)
                                n470 = Divide(x=1.0 ("Digital DC (%)"), y=w2734) -> (x/y=w2733:dbl)
                                n471 = Multiply(x=100.0, y=w2733) -> (x*y=w2732:dbl)
                                n472 = Divide(x=w2739, y=w2734) -> (x/y=w2737:dbl)
                                n473 = call "replace DO wf param.vi"("Digital Freq (Hz)"=w2737, "Digital DC (%)"=w2732, "Digital phase"=w2744, "Sampling frequency (Hz)"=w2738, "Digital time offset (s)"=w2744, "index of DO wave"=w2736, "padding value"=w2744, "matlab wave file"=path "LT" ("matlab wave number")) -> ()  [unwired: 3 in]
                                }
                                }
                                }
                                }
                                n474 = Build Array(w2720) -> (w2719:T17)
                                }
                                }
                              }
                              frame #9 {
                                n475 = Build Array(w2749, w2748) -> (w2751:bool[])
                                n476 = Boolean Array To Number(Boolean array=w2751) -> (number=w2750:u32)
                                n477 = case shown="2" w2750 {
                                tunnel: w2747 -> [_ w2803 _ w2807]
                                tunnel: [_ w2798 _ w2804] -> w2746
                                frame 1 {
                                n478 = call "2pparameters.vi"("command"="get") -> ("params out"=w2758:T10)  [unwired: 1 in]
                                n479 = Unbundle By Name(w2758) -> ("wavdet"=w2759:bool, "sAOxy"=w2761:i32, "refwfsize"=w2762:dbl, "srate Img"=w2760:sgl)
                                n480 = call "waveformsDObuffer.vi"("command"="get") -> ("DO wf out"=w2754:digitalwaveform[])  [unwired: 1 in]
                                n481 = case shown="True" w2759 {
